vi "Create_SaveFile.vi"(7 "File Header Format":string, 8 "error in":errorcluster, 9 "Operation Type":string, 11 "Template File":path) -> (0 "error out":errorcluster, 3 "refnum out":refnum<file>)   [LabVIEW 2010]
doc: "This VI creates a text file to be used to save data from the application. The file is created from a template file that contains the user specified comments and is opened, operation type appended, and reference to the file returned.\n\nInputs:\nFile Header Format - (str) Format of header string to append to file\nTemplate File - (path) path to the template file used to create the desired file\nOperation Type - (str) type of operation whose information is being saved (also appended into the file)\nerror in - error input cluster\n\nOutputs:\nrefnum out - (refnum) reference to the file to be written to. NOTE: the reference should be closed when manipulation/writing is completed.\nerror out - error output cluster"
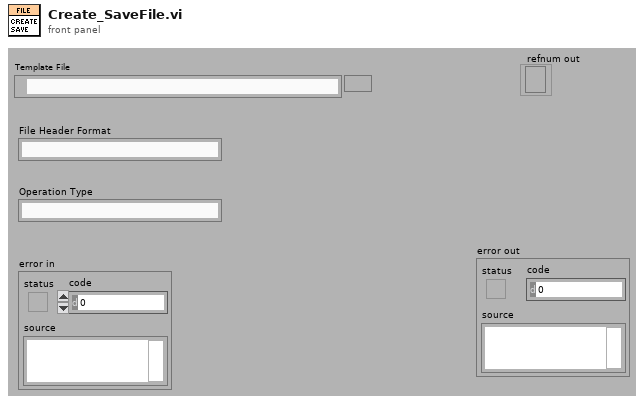
[diagram p1: front panel]
types:
  T1 = enum16{"open", "replace", "create", "open or create", "replace or create", "replace or create with confirmation"}
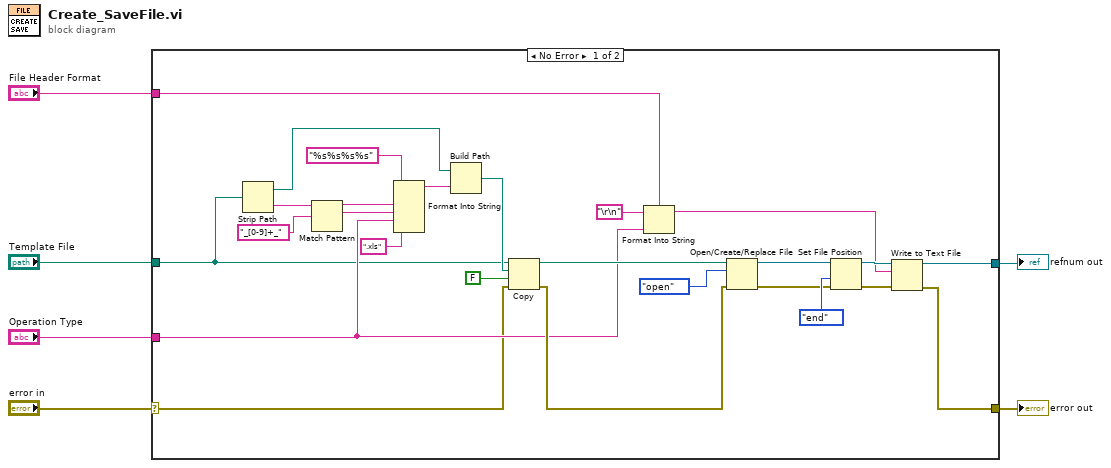
[diagram p0: block diagram]
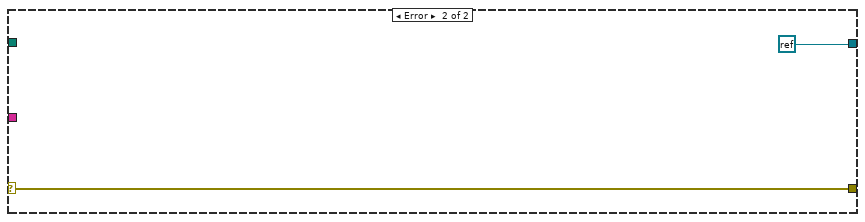
[diagram p2: hidden frame]
diagram:
  n1 = case shown="No Error" "error in" {
    selector: "error in" -> [w8 w34]
    tunnel: "File Header Format" -> [w28 _]
    tunnel: "Operation Type" -> [w27 _]
    tunnel: "Template File" -> [w17 _]
    tunnel: [w11 refnum<k0> refnum] -> w3
    tunnel: [w10 w34] -> w2
    frame No Error {
      n2 = Strip Path(path=w17) -> (stripped path=w23:path, name=w18:string)
      n3 = Match Pattern(string=w18, regular expression="_[0-9]+_") -> (before substring=w20:string, match substring=w22:string)  [unwired: 3 out]
      n4 = Format Into String(format string="%s%s%s%s", w20, w22, w27, ".xls" ("input 4")) -> (resulting string=w24:string)  [unwired: 2 in, 1 out]
      n5 = Build Path(base path=w23, name or relative path=w24) -> (appended path=w25:path)
      n6 = Copy(8:w8, 9:FALSE ("overwrite (F)"), 10:w25, 11:w17) -> (0:w32:errorcluster, 3:w31:path)  [unwired: 2 out]
      n7 = Format Into String(format string=w28, initial string="\r\n", w27) -> (resulting string=w9:string)  [unwired: 1 in, 1 out]
      n8 = Open/Create/Replace File(file path (use dialog)=w31, error in=w32, operation (0:open)=T1."open") -> (refnum out=w13:refnum<file>, error out=w12:errorcluster)  [unwired: 4 out]
      n9 = Set File Position(refnum=w13, from (0:start)=enum16{"start", "end", "current"}."end", error in=w12) -> (refnum out=w15:refnum<file>, error out=w16:errorcluster)  [unwired: 1 out]
      n10 = Write to Text File(file (use dialog)=w15, text=w9, error in=w16) -> (refnum out=w11:refnum<file>, error out=w10:errorcluster)  [unwired: 2 out]
    }
    frame Error {
    }
  }
  "error out" <- w2
  "refnum out" <- w3
